vi "25_P-GPIB-LockIn510.vi"(0 "P-LockIn":string="23", 1 "P-DMM":string="16", 2 "Lecturas":i32=1, 3 "error in (no error)":errorcluster, 4 "Tipo":u16(ring) items=["LockIn", "LockIn-DMM"]) -> (5 "LockIn":dbl=-0.0002, 6 "DMM":dbl, 7 "error out":errorcluster)   [LabVIEW 2018]
uses:
  <vilib>/Utility/error.llb/DialogType.ctl
panel:
  out "Cont-C":i32=1
  out "Cont-B":i32=50
  out "Cont-A":i32=50
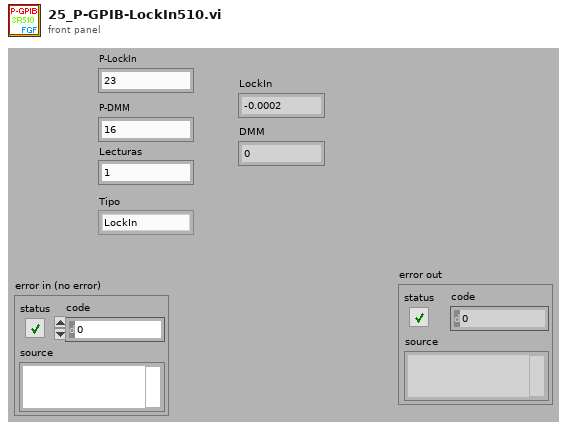
[diagram p1: front panel]
types:
  T1 = typedef "DialogType.ctl" = u16
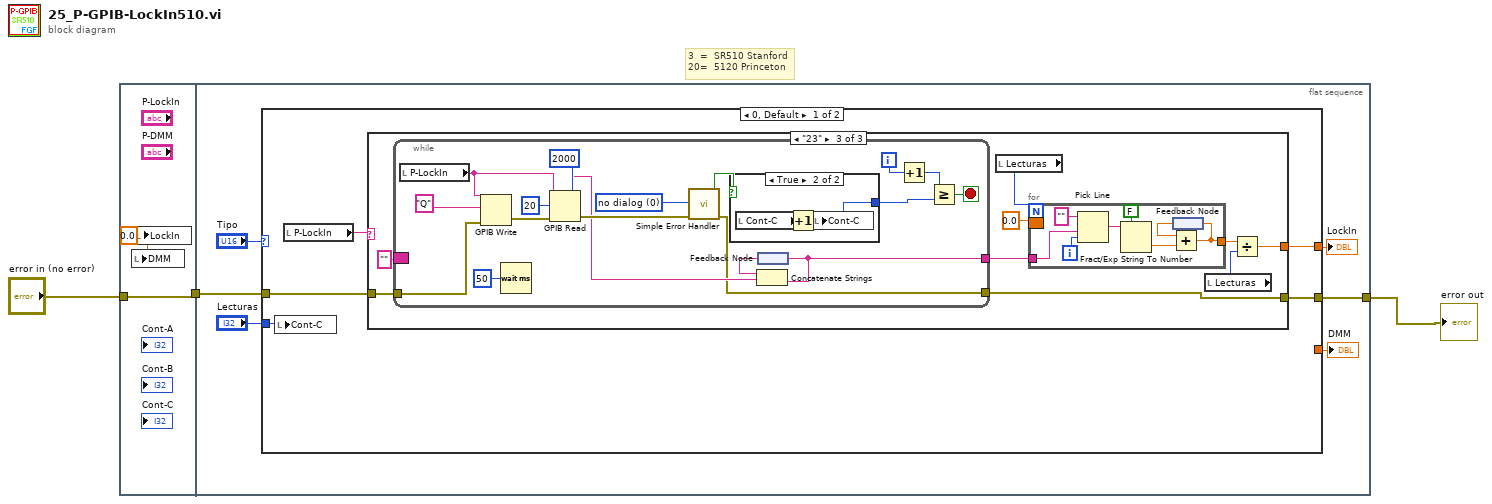
[diagram p0: block diagram]
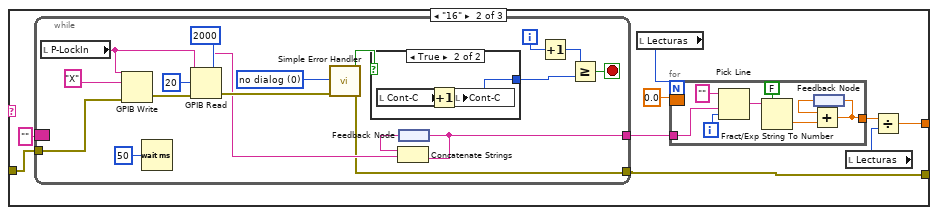
[diagram p3: hidden frame]
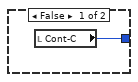
[diagram p4: hidden frame]
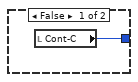
[diagram p5: hidden frame]
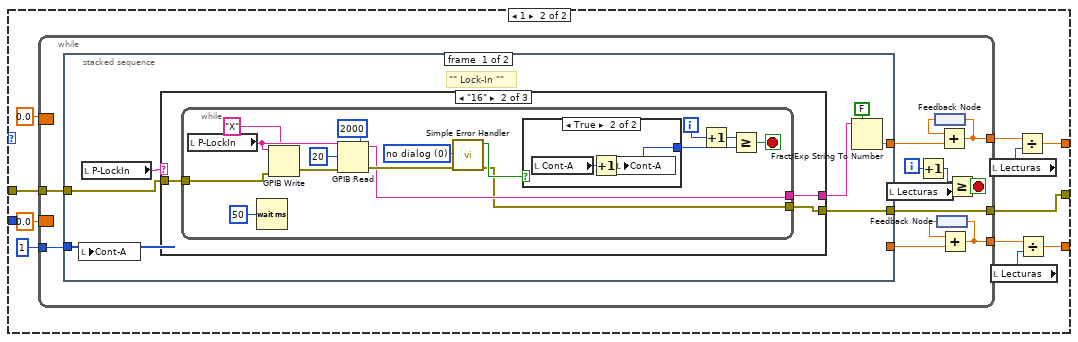
[diagram p6: hidden frame]
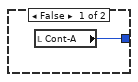
[diagram p8: hidden frame]
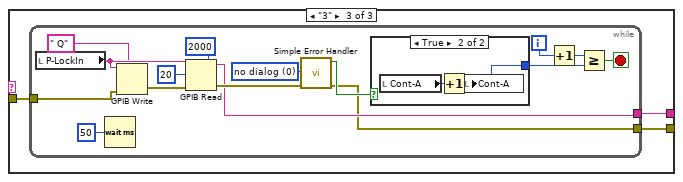
[diagram p9: hidden frame]
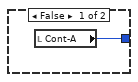
[diagram p10: hidden frame]
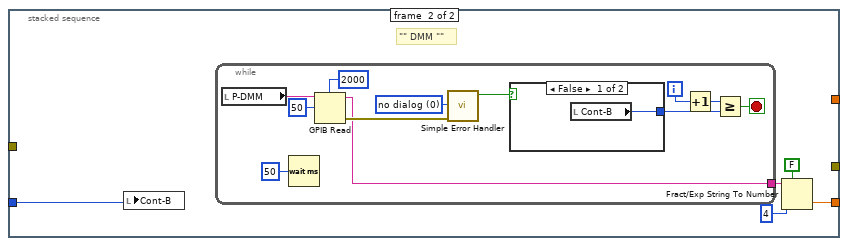
[diagram p11: hidden frame]
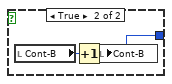
[diagram p12: hidden frame]
diagram:
  # "3  =  SR510 Stanford\n20=  5120 Princeton"
  n1 = flat-sequence {
    tunnel: [w4] -> w3
    tunnel: "error in (no error)" -> [w4]
    tunnel: w3 -> [w7]
    tunnel: [w6] -> w1
    frame #0 {
      w5 = 0.0 ("LockIn")
      n2 = local write "DMM"(w5) -> ()
      n3 = local write "LockIn"(w5) -> ()
    }
    frame #1 {
      n4 = case shown="0, Default" "Tipo" {
        tunnel: [w16 w99] -> w11
        tunnel: [_ w98] -> w10
        tunnel: "Lecturas" -> [w15 _]
        tunnel: w7 -> [w13 w95]
        tunnel: [w12 w94] -> w6
        frame 0, Default {
          n5 = local write "Cont-C"(w15) -> ()
          n6 = local read "P-LockIn"() -> (w14:string)
          n7 = case shown="\"23\"" w14 {
            tunnel: [_ w20 w58] -> w16
            tunnel: w13 -> [w17 w19 w57]
            tunnel: [w17 w18 w56] -> w12
            frame "False", Default {
            }
            frame "16" {
              n8 = while {
                border: "" -> [_]
                tunnel: [w40] -> w26
                tunnel: w19 -> [w36]
                tunnel: [w35] -> w18
                i -> [w52]
                stop <- w49 stop-if-true
                w44 = T1 0 items=["no dialog", "OK message", "continue or stop message", "OK message + warnings", "continue/stop + warnings"] ("type of dialog (OK msg:1)")
                n9 = local read "P-LockIn"() -> (w41:string)
                n10 = GPIB Write(0:w41, 1:"X" ("Write"), 3:w36) -> (6:w46:errorcluster)  [unwired: 2 in, 1 out]
                n11 = Wait (ms)(milliseconds to wait=u32 50) -> ()  [unwired: 1 out]
                n12 = GPIB Read(0:w41, 1:20 ("# Bytes to Read"), 3:w46, 4:2000 ("timeout ms (488.2 global)")) -> (5:w38:string, 7:w43:errorcluster)  [unwired: 1 in, 1 out]
                n13 = call <vilib>:"Simple Error Handler.vi"("type of dialog (OK msg:1)"=w44, "error in (no error)"=w43) -> ("error?"=w39:bool, "error out"=w35:errorcluster)  [unwired: 3 in, 3 out]
                n14 = case shown="True" w39 {
                  tunnel: [w53 w54] -> w51
                  frame False {
                    n15 = local read "Cont-C"() -> (w53:i32)
                  }
                  frame True {
                    n16 = local read "Cont-C"() -> (w55:i32)
                    n17 = Increment(x=w55) -> (x+1=w54:i32)
                    n18 = local write "Cont-C"(w54) -> ()
                  }
                }
                n19 = feedback #1() -> (w42:string)
                n20 = Concatenate Strings(w42, w38) -> (w40:string)
                n21 = feedback-in #1(w40) -> ()
                n22 = Increment(x=w52) -> (x+1=w50:i32)
                n23 = Greater Or Equal?(x=w50, y=w51) -> (x >= y?=w49:bool)
              }
              n24 = local read "Lecturas"() -> (w24:i32)
              n25 = for {
                N: w24 -> [_]
                border: 0.0 -> [_]
                tunnel: [w30] -> w23
                tunnel: w26 -> [w29]
                i -> [w34]
                n26 = Pick Line(string ("")="", multi-line string=w29, line index=w34) -> (output string=w28:string)
                n27 = Fract/Exp String To Number(use system decimal point (T)=FALSE, string=w28) -> (number=w27:dbl)  [unwired: 2 in, 1 out]
                n28 = feedback #2() -> (w31:dbl)
                n29 = Add(x=w31, y=w27) -> (x+y=w30:dbl)
                n30 = feedback-in #2(w30) -> ()
              }
              n31 = local read "Lecturas"() -> (w22:i32)
              n32 = Divide(x=w23, y=w22) -> (x/y=w20:dbl)
            }
            frame "23" {
              n33 = while {
                border: "" -> [_]
                tunnel: [w78] -> w64
                tunnel: w57 -> [w74]
                tunnel: [w73] -> w56
                i -> [w90]
                stop <- w87 stop-if-true
                w82 = T1 0 items=["no dialog", "OK message", "continue or stop message", "OK message + warnings", "continue/stop + warnings"] ("type of dialog (OK msg:1)")
                n34 = local read "P-LockIn"() -> (w79:string)
                n35 = GPIB Write(0:w79, 1:"Q" ("Write"), 3:w74) -> (6:w84:errorcluster)  [unwired: 2 in, 1 out]
                n36 = Wait (ms)(milliseconds to wait=u32 50) -> ()  [unwired: 1 out]
                n37 = GPIB Read(0:w79, 1:20 ("# Bytes to Read"), 3:w84, 4:2000 ("timeout ms (488.2 global)")) -> (5:w76:string, 7:w81:errorcluster)  [unwired: 1 in, 1 out]
                n38 = call <vilib>:"Simple Error Handler.vi"("type of dialog (OK msg:1)"=w82, "error in (no error)"=w81) -> ("error?"=w77:bool, "error out"=w73:errorcluster)  [unwired: 3 in, 3 out]
                n39 = case shown="True" w77 {
                  tunnel: [w91 w92] -> w89
                  frame False {
                    n40 = local read "Cont-C"() -> (w91:i32)
                  }
                  frame True {
                    n41 = local read "Cont-C"() -> (w93:i32)
                    n42 = Increment(x=w93) -> (x+1=w92:i32)
                    n43 = local write "Cont-C"(w92) -> ()
                  }
                }
                n44 = feedback #3() -> (w80:string)
                n45 = Concatenate Strings(w80, w76) -> (w78:string)
                n46 = feedback-in #3(w78) -> ()
                n47 = Increment(x=w90) -> (x+1=w88:i32)
                n48 = Greater Or Equal?(x=w88, y=w89) -> (x >= y?=w87:bool)
              }
              n49 = local read "Lecturas"() -> (w62:i32)
              n50 = for {
                N: w62 -> [_]
                border: 0.0 -> [_]
                tunnel: [w68] -> w61
                tunnel: w64 -> [w67]
                i -> [w72]
                n51 = Pick Line(string ("")="", multi-line string=w67, line index=w72) -> (output string=w66:string)
                n52 = Fract/Exp String To Number(use system decimal point (T)=FALSE, string=w66) -> (number=w65:dbl)  [unwired: 2 in, 1 out]
                n53 = feedback #4() -> (w69:dbl)
                n54 = Add(x=w69, y=w65) -> (x+y=w68:dbl)
                n55 = feedback-in #4(w68) -> ()
              }
              n56 = local read "Lecturas"() -> (w60:i32)
              n57 = Divide(x=w61, y=w60) -> (x/y=w58:dbl)
            }
          }
        }
        frame 1 {
          n58 = while {
            border: 0.0 -> [_]
            tunnel: 1 ("Cont-A") -> [w114]
            border: 0.0 -> [_]
            tunnel: [w108] -> w100
            tunnel: [w111] -> w97
            tunnel: w95 -> [w106]
            tunnel: [w105] -> w94
            i -> [w115]
            stop <- w116 stop-if-true
            n59 = stacked-sequence {
              tunnel: w114 -> [w121 w171]
              tunnel: [w122 _] -> w107
              tunnel: [_ w172] -> w112
              tunnel: w106 -> [w119 _]
              tunnel: [w118 _] -> w105
              frame #0 {
                # "\"\" Lock-In \"\""
                n60 = local write "Cont-A"(w121) -> ()
                n61 = local read "P-LockIn"() -> (w120:string)
                n62 = case shown="\"16\"" w120 {
                  tunnel: [_ w128 w150] -> w123
                  tunnel: w119 -> [w125 w127 w149]
                  tunnel: [w125 w126 w148] -> w118
                  frame "False", Default {
                  }
                  frame "16" {
                    n63 = while {
                      tunnel: [w132] -> w128
                      tunnel: w127 -> [w130]
                      tunnel: [w129] -> w126
                      i -> [w144]
                      stop <- w141 stop-if-true
                      w138 = T1 0 items=["no dialog", "OK message", "continue or stop message", "OK message + warnings", "continue/stop + warnings"] ("type of dialog (OK msg:1)")
                      n64 = local read "P-LockIn"() -> (w140:string)
                      n65 = Wait (ms)(milliseconds to wait=u32 50) -> ()  [unwired: 1 out]
                      n66 = GPIB Write(0:w140, 1:"X" ("Write"), 3:w130) -> (6:w136:errorcluster)  [unwired: 2 in, 1 out]
                      n67 = GPIB Read(0:w140, 1:20 ("# Bytes to Read"), 3:w136, 4:2000 ("timeout ms (488.2 global)")) -> (5:w132:string, 7:w139:errorcluster)  [unwired: 1 in, 1 out]
                      n68 = call <vilib>:"Simple Error Handler.vi"("type of dialog (OK msg:1)"=w138, "error in (no error)"=w139) -> ("error?"=w133:bool, "error out"=w129:errorcluster)  [unwired: 3 in, 3 out]
                      n69 = case shown="True" w133 {
                        tunnel: [w145 w146] -> w143
                        frame False {
                          n70 = local read "Cont-A"() -> (w145:i32)
                        }
                        frame True {
                          n71 = local read "Cont-A"() -> (w147:i32)
                          n72 = Increment(x=w147) -> (x+1=w146:i32)
                          n73 = local write "Cont-A"(w146) -> ()
                        }
                      }
                      n74 = Increment(x=w144) -> (x+1=w142:i32)
                      n75 = Greater Or Equal?(x=w142, y=w143) -> (x >= y?=w141:bool)
                    }
                  }
                  frame "3" {
                    n76 = while {
                      tunnel: [w154] -> w150
                      tunnel: w149 -> [w152]
                      tunnel: [w151] -> w148
                      i -> [w166]
                      stop <- w163 stop-if-true
                      w160 = T1 0 items=["no dialog", "OK message", "continue or stop message", "OK message + warnings", "continue/stop + warnings"] ("type of dialog (OK msg:1)")
                      n77 = local read "P-LockIn"() -> (w162:string)
                      n78 = Wait (ms)(milliseconds to wait=u32 50) -> ()  [unwired: 1 out]
                      n79 = GPIB Write(0:w162, 1:" Q" ("Write"), 3:w152) -> (6:w158:errorcluster)  [unwired: 2 in, 1 out]
                      n80 = GPIB Read(0:w162, 1:20 ("# Bytes to Read"), 3:w158, 4:2000 ("timeout ms (488.2 global)")) -> (5:w154:string, 7:w161:errorcluster)  [unwired: 1 in, 1 out]
                      n81 = call <vilib>:"Simple Error Handler.vi"("type of dialog (OK msg:1)"=w160, "error in (no error)"=w161) -> ("error?"=w155:bool, "error out"=w151:errorcluster)  [unwired: 3 in, 3 out]
                      n82 = case shown="True" w155 {
                        tunnel: [w167 w168] -> w165
                        frame False {
                          n83 = local read "Cont-A"() -> (w167:i32)
                        }
                        frame True {
                          n84 = local read "Cont-A"() -> (w169:i32)
                          n85 = Increment(x=w169) -> (x+1=w168:i32)
                          n86 = local write "Cont-A"(w168) -> ()
                        }
                      }
                      n87 = Increment(x=w166) -> (x+1=w164:i32)
                      n88 = Greater Or Equal?(x=w164, y=w165) -> (x >= y?=w163:bool)
                    }
                  }
                }
                n89 = Fract/Exp String To Number(use system decimal point (T)=FALSE, string=w123) -> (number=w122:dbl)  [unwired: 2 in, 1 out]
              }
              frame #1 {
                # "\"\" DMM \"\""
                n90 = local write "Cont-B"(w171) -> ()
                n91 = while {
                  tunnel: [w176] -> w173
                  i -> [w186]
                  stop <- w183 stop-if-true
                  w180 = T1 0 items=["no dialog", "OK message", "continue or stop message", "OK message + warnings", "continue/stop + warnings"] ("type of dialog (OK msg:1)")
                  n92 = local read "P-DMM"() -> (w178:string)
                  n93 = Wait (ms)(milliseconds to wait=u32 50) -> ()  [unwired: 1 out]
                  n94 = GPIB Read(0:w178, 1:50 ("# Bytes to Read"), 4:2000 ("timeout ms (488.2 global)")) -> (5:w176:string, 7:w179:errorcluster)  [unwired: 2 in, 1 out]
                  n95 = call <vilib>:"Simple Error Handler.vi"("type of dialog (OK msg:1)"=w180, "error in (no error)"=w179) -> ("error?"=w177:bool)  [unwired: 3 in, 4 out]
                  n96 = case shown="False" w177 {
                    tunnel: [w187 w188] -> w185
                    frame False {
                      n97 = local read "Cont-B"() -> (w187:i32)
                    }
                    frame True {
                      n98 = local read "Cont-B"() -> (w189:i32)
                      n99 = Increment(x=w189) -> (x+1=w188:i32)
                      n100 = local write "Cont-B"(w188) -> ()
                    }
                  }
                  n101 = Increment(x=w186) -> (x+1=w184:i32)
                  n102 = Greater Or Equal?(x=w184, y=w185) -> (x >= y?=w183:bool)
                }
                n103 = Fract/Exp String To Number(use system decimal point (T)=FALSE, string=w173, offset=4) -> (number=w172:dbl)  [unwired: 1 in, 1 out]
              }
            }
            n104 = local read "Lecturas"() -> (w110:i32)
            n105 = Increment(x=w115) -> (x+1=w109:i32)
            n106 = feedback #5() -> (w117:dbl)
            n107 = feedback #6() -> (w113:dbl)
            n108 = Add(x=w117, y=w107) -> (x+y=w108:dbl)
            n109 = feedback-in #5(w108) -> ()
            n110 = Add(x=w113, y=w112) -> (x+y=w111:dbl)
            n111 = feedback-in #6(w111) -> ()
            n112 = Greater Or Equal?(x=w109, y=w110) -> (x >= y?=w116:bool)
          }
          n113 = local read "Lecturas"() -> (w102:i32)
          n114 = local read "Lecturas"() -> (w101:i32)
          n115 = Divide(x=w100, y=w102) -> (x/y=w99:dbl)
          n116 = Divide(x=w97, y=w101) -> (x/y=w98:dbl)
        }
      }
      "LockIn" <- w11
      "DMM" <- w10
    }
  }
  "error out" <- w1
